vi "Test Append To Empty Test Suite.vi"(8 "error in (no error)":errorcluster, 11 "LUnit Test Suite Tests In":refnum<class "LUnit Test Suite Tests.lvclass">) -> (0 "error out":errorcluster, 3 "LUnit Test Suite Tests Out":refnum<class "LUnit Test Suite Tests.lvclass">)   [LabVIEW 2020, in "LUnit Test Suite Tests.lvclass"]
uses:
  LUnit Test Suite Tests.lvclass
  C:/Program Files (x86)/National Instruments/LabVIEW 2020/vi.lib/Astemes/LUnit/Test Case.lvclass
  LUnit Test Suite/LUnit Test Suite V2.lvclass
  C:/Git/astemes-lunit/source/Rewrite Project/Run/Runnable.lvclass
  Light Test Case Double/Light Test Case Double.lvclass
  C:/Git/astemes-lunit/source/Rewrite Project/LUnit Test Case/LUnit Test Case V2.lvclass
  Result/Type.ctl
  <vilib>/Astemes/LUnit/Test Case.lvclass/Test Case.ctl
  b74e4934-f044-4222-b3dd-fc90e6c1bd4f.vi
  <vilib>/Astemes/LUnit/Palette/Pass.vi
  <vilib>/Astemes/LUnit/Palette/Fail.vi
  <vilib>/Astemes/LUnit/Compare Variants.vi
  <vilib>/Astemes/LUnit/Describe Comparison.vi
  <vilib>/Astemes/LUnit/Set Assertion Type.vi
  <vilib>/Astemes/LUnit/Add test result.vi
  <vilib>/Astemes/LUnit/Variant to string.vi
  <vilib>/Astemes/LUnit/LUnit Record Assertion Result.vi
  <vilib>/Astemes/LUnit/LUnit Aggregate Assertion Results.vi
  <vilib>/Astemes/LUnit/Method Result/LUnit Merge Status.vi
  <vilib>/Astemes/LUnit/LUnit Concatenate result strings.vi
  <vilib>/Utility/Data Type/Get Type Information.vi
  <vilib>/Utility/LVClass/Get LV Class Name.vi
  Result/Result.lvlib
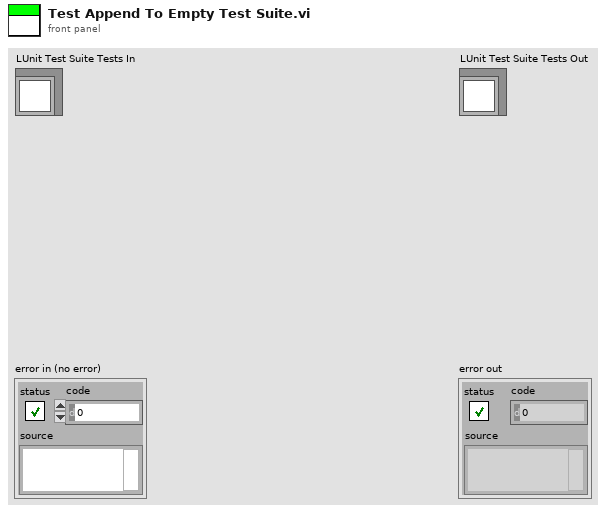
[diagram p1: front panel]
types:
  T1 = typedef "Result.lvlib/Result.ctl" = cluster{"Case":string, "Message":string, "Description":string, "Status":T2, "Result Type":T3, "Execution Time":dbl}
  T2 = typedef "Result.lvlib/Status.ctl" = enum16{"Passed", "Failed", "Error", "Skipped", "Setup Error", "Broken", "Teardown Error"}
  T3 = typedef "Result.lvlib/Type.ctl" = enum16{"Method", "Case", "Suite", "Pass", "Fail", "Skip", "Pass if", "Fail if", "Pass if Error", "Fail if Error", "Pass if Equal", "Fail if Equal"}
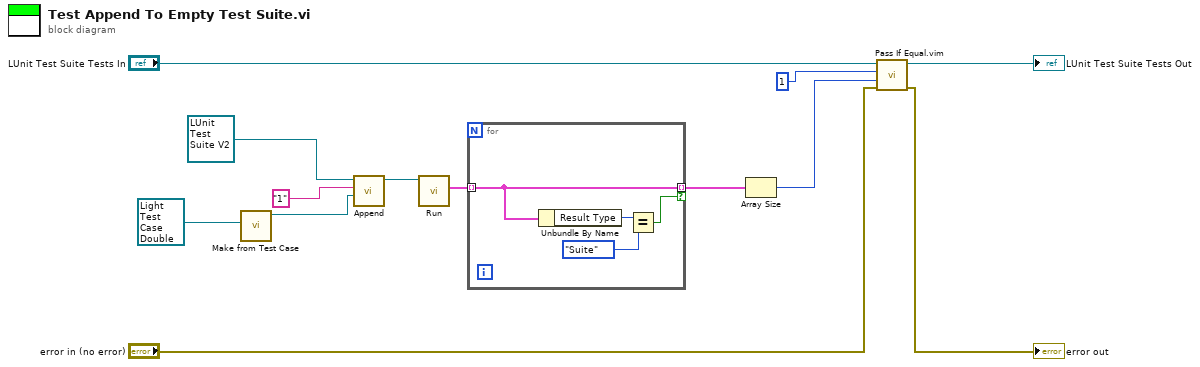
[diagram p0: block diagram]
diagram:
  n1 = call "Make from Test Case.vi"("LUnit Test Case"=refnum<class "Light Test Case Double.lvclass"> refnum ("Light Test Case Double.lvclass")) -> ("LUnit Test Suite V2 out"=w5:refnum<class "LUnit Test Suite V2.lvclass">)  [unwired: 9 in, 1 out]
  n2 = call "Append.vi"("Runnable"=w5, "Name"="1", "LUnit Test Suite V2 in"=refnum<class "LUnit Test Suite V2.lvclass"> refnum ("Run in")) -> ("LUnit Test Suite V2 out"=w7:refnum<class "LUnit Test Suite V2.lvclass">)  [unwired: 7 in, 1 out]
  n3 = call-dynamic "Run.vi"("Run in"=w7) -> ("Results"=w3:T1[])  [unwired: 9 in, 1 out]
  n4 = for {
    tunnel: w3 -> [w15] mode=indexing
    tunnel: [w15] -> w2 mode=indexing if=w14
    n5 = Unbundle By Name(w15) -> ("Result Type"=w17:T3)
    n6 = Equal?(x=w17, y=Type."Suite") -> (x = y?=w14:bool)
  }
  n7 = Array Size(array=w2) -> (size(s)=w9:i32)
  n8 = call "Pass If Equal.vim"("error in (no error)"="error in (no error)", "Actual"=w9, "Expected"=1 ("size(s)"), "LUnit Test Case In"="LUnit Test Suite Tests In") -> ("error out"=→"error out":errorcluster, "LUnit Test Case Out"=→"LUnit Test Suite Tests Out":refnum<class "LUnit Test Suite Tests.lvclass">)  [unwired: 6 in]
